vi "Poll Door Status.vi"(8 "error in (no error)":errorcluster, 11 "task/channels in":refnum<k21>) -> (0 "error out":errorcluster, 1 "Cable":bool, 2 "Door Status":bool, 3 "task out":refnum<k21>)   [LabVIEW 2018]
uses:
  <vilib>/DAQmx/read.llb/DAQmx Read (Digital 2D Bool NChan 1Samp NLine).vi
  <vilib>/DAQmx/miscellaneous.llb/DAQmx Fill In Error Info.vi
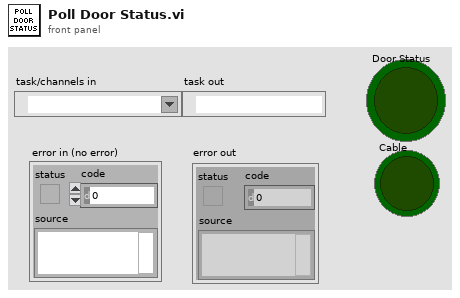
[diagram p1: front panel]
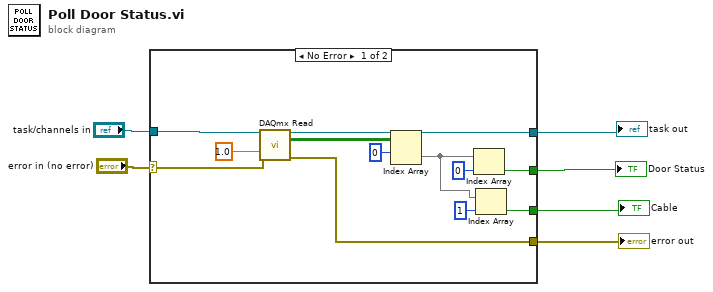
[diagram p0: block diagram]
diagram:
  n1 = case shown="No Error" "error in (no error)" {
    selector: "error in (no error)" -> [w14 w19]
    tunnel: [w18 w19] -> w6
    tunnel: [w16 w20] -> w5
    tunnel: "task/channels in" -> [w15 w20]
    tunnel: [w10 _] -> w2
    tunnel: [w7 _] -> w1
    frame No Error {
      n2 = call-poly <vilib>:"DAQmx Read.vi"("task/channels in"=w15, "timeout"=1.0, "error in"=w14) -> ("task out"=w16:refnum<k21>, "data"=w13:bool[][], "error out"=w18:errorcluster)  [unwired: 10 in]
      n3 = Index Array(array=w13, index (row)=0) -> (element=w8:bool[])  [unwired: 1 in]
      n4 = Index Array(array=w8, index=0) -> (element=w10:bool)
      n5 = Index Array(array=w8, index=1) -> (element=w7:bool)
    }
    frame Error {
    }
  }
  "Door Status" <- w2
  "error out" <- w6
  "task out" <- w5
  "Cable" <- w1
